vi "SwerveDriveSystem.vi"(4 "Enable Auto Swerve Drive":bool, 5 "Automatic State Control Mode (F)":bool, 6 "Robot Motion Commands":T1, 7 "Robot field orientation (deg)":dbl, 8 "Drive Joystick Buttons":T4, 9 "Turn":dbl, 10 "Forward":dbl, 11 "Right":dbl) -> ()   [LabVIEW 2019]
uses:
  Controls/DriveJoystickData.ctl
  Controls/Robot Pivot Motion Commands.ctl
  Controls/Pivot Motor Commands.ctl
  Controls/Robot Drive Mode.ctl
  Global Variables/reset gyro.vi
  <vilib>/Rock Robotics/Network Tables/NT Read Numeric Array.vi
  <vilib>/Rock Robotics/Network Tables/NT Write Boolean.vi
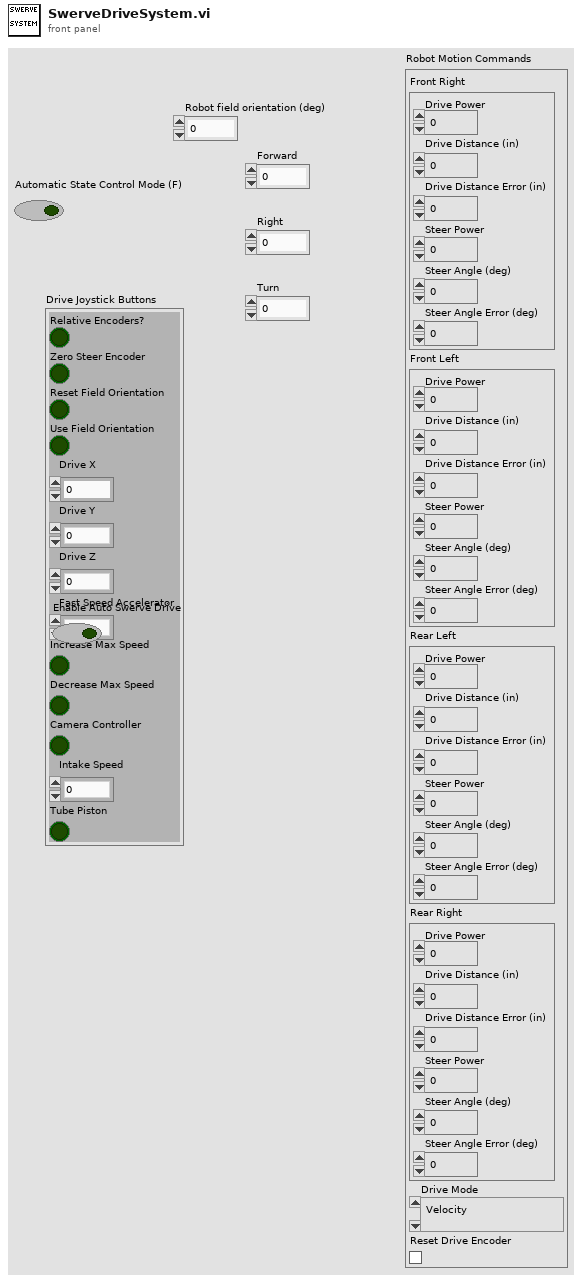
[diagram p1: front panel]
types:
  T1 = typedef "Robot Pivot Motion Commands.ctl" = cluster{"Front Right":T2, "Front Left":T2, "Rear Left":T2, "Rear Right":T2, "Drive Mode":T3, "Reset Drive Encoder":bool}
  T2 = typedef "Pivot Motor Commands.ctl" = cluster{"Drive Power":dbl, "Drive Distance (in)":dbl, "Drive Distance Error (in)":dbl, "Steer Power":dbl, "Steer Angle (deg)":dbl, "Steer Angle Error (deg)":dbl}
  T3 = typedef "Robot Drive Mode.ctl" = enum16{"Velocity", "Distance"}
  T4 = typedef "DriveJoystickData.ctl" = cluster{"Relative Encoders?":bool, "Zero Steer Encoder":bool, "Reset Field Orientation":bool, "Use Field Orientation":bool, "Drive X":dbl, "Drive Y":dbl, "Drive Z":dbl, "Fast Speed Accelerator":dbl, "Increase Max Speed":bool, "Decrease Max Speed":bool, "Camera Controller":bool, "Intake Speed":dbl, "Tube Piston":bool}
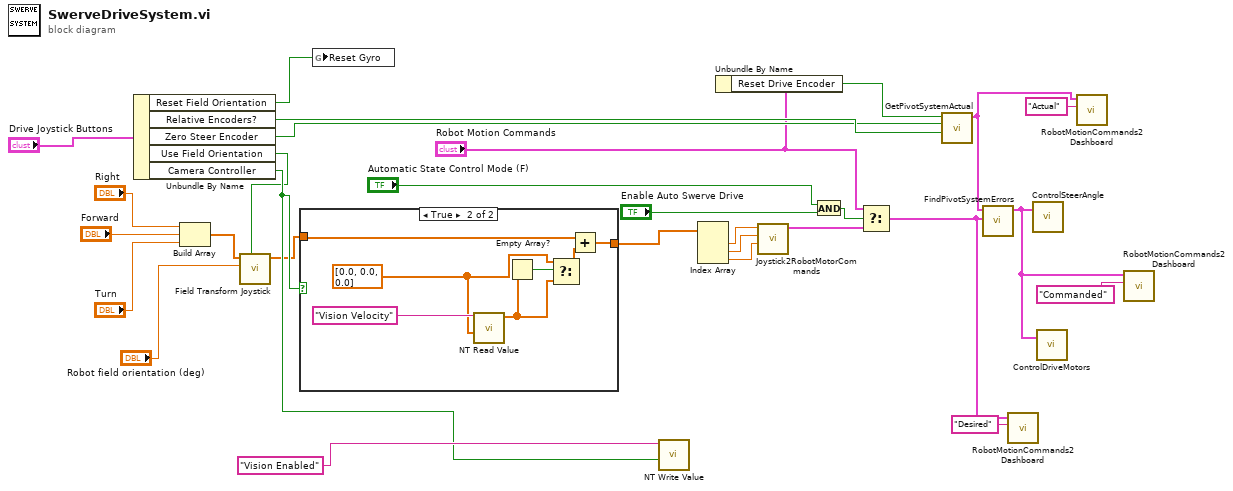
[diagram p0: block diagram]
diagram:
  n1 = Unbundle By Name("Drive Joystick Buttons") -> ("Reset Field Orientation"=w23:bool, "Relative Encoders?"=w21:bool, "Zero Steer Encoder"=w20:bool, "Use Field Orientation"=w4:bool, "Camera Controller"=w5:bool)
  n2 = Build Array("Right", "Forward", "Turn") -> (w24:dbl[])
  n3 = call "Field Transform Joystick.vi"("use field orientation"=w4, "robot field orientation (deg)"="Robot field orientation (deg)", "Joystick Values"=w24) -> ("Transformed Joystick Values"=w2:dbl[])  [unwired: 8 in]
  n4 = case shown="True" w5 {
    tunnel: w2 -> [w30 w31]
    tunnel: [w30 w32] -> w1
    frame False {
    }
    frame True {
      w35 = dbl[] [0.0, 0.0, 0.0] ("Default Value")
      n5 = call-poly <vilib>:"NT Read Value.vi"("Default Value"=w35, "Name"="Vision Velocity") -> ("Numeric Array"=w34:dbl[])  [unwired: 8 in, 1 out]
      n6 = Empty Array?(array=w34) -> (empty?=w36:bool)
      n7 = Select(t=w35, s=w36, f=w34) -> (s? t:f=w33:dbl[])
      n8 = Add(x=w31, y=w33) -> (x+y=w32:dbl[])
    }
  }
  n9 = global write "reset gyro.vi" "Reset Gyro"(w23) -> ()
  n10 = call-poly <vilib>:"NT Write Value.vi"("Boolean"=w5, "Name"="Vision Enabled") -> ()  [unwired: 9 in, 1 out]
  n11 = Index Array(array=w1) -> (element #1=w29:dbl, element #2=w28:dbl, element #3=w7:dbl)  [unwired: 3 in]
  n12 = Unbundle By Name("Robot Motion Commands") -> ("Reset Drive Encoder"=w9:bool)
  n13 = call "Joystick2RobotMotorCommands.vi"("Joystick R"=w7, "Joystick Y"=w28, "Joystick X"=w29) -> ("Robot Motion Commands"=w22:T1)  [unwired: 8 in]
  n14 = And(x="Automatic State Control Mode (F)", y="Enable Auto Swerve Drive") -> (x .and. y?=w11:bool)
  n15 = Select(t="Robot Motion Commands", s=w11, f=w22) -> (s? t:f=w19:T1)
  n16 = call "GetPivotSystemActual.vi"("Relative Encoders?"=w21, "Zero Relative Encoder"=w20, "Zero Drive Encoder"=w9) -> ("Robot Motion Commands Out"=w16:T1)  [unwired: 8 in]
  n17 = call "FindPivotSystemErrors.vi"("Desired Motion"=w19, "Actual Pivot System"=w16) -> ("Commanded Motion"=w14:T1)  [unwired: 9 in]
  n18 = call "RobotMotionCommands2Dashboard.vi"("Label"="Desired", "Robot Motion Commands"=w19) -> ()  [unwired: 10 in]
  n19 = call "ControlSteerAngle.vi"("Robot Motion Commands"=w14) -> ()  [unwired: 1 in, 1 out]
  n20 = call "ControlDriveMotors.vi"("Robot Motion Commands"=w14) -> ()  [unwired: 2 in]
  n21 = call "RobotMotionCommands2Dashboard.vi"("Label"="Actual", "Robot Motion Commands"=w16) -> ()  [unwired: 10 in]
  n22 = call "RobotMotionCommands2Dashboard.vi"("Label"="Commanded", "Robot Motion Commands"=w14) -> ()  [unwired: 10 in]
